vi "Var_señales_G2.vi"() -> ()   [LabVIEW 2018]
panel:
  in  "Var_V_G2":sgl
  in  "Var_Frec_G2":sgl
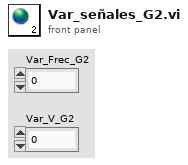
[diagram p1: front panel]
diagram:
